vi "UIGetFlaggedRefs.vi"(6 "Check Flag (T)":bool=TRUE, 8 "error in":errorcluster, 10 "Flag":string, 11 "Control in":refnum<vi>) -> (0 "error out":errorcluster, 1 "UI Ctrl DataType":T1[](array[typedef]), 2 "UI Ctrl Names":string[](array[string]), 3 "UI Ctrl Refs":refnum<vi>[](array[refnum]))   [LabVIEW 2025, in "UI_Library.lvlib" / "UI_Library.lvclass"]
doc: "Get Control and subControls info"
uses:
  UI_Library.lvclass
  <vilib>/Utility/Data Type/Type Definitions/Data Type.ctl
  <vilib>/Utility/Data Type/NI_Data Type.lvlib
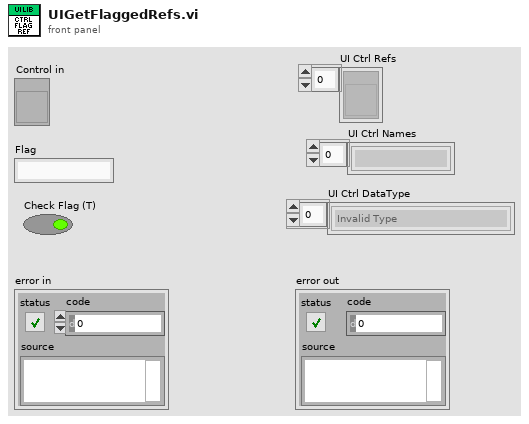
[diagram p1: front panel]
types:
  T1 = typedef "NI_Data Type.lvlib/Data Type.ctl" = enum8{"Invalid Type", "Void", "I8", "I16", "I32", "I64", "U8", "U16", "U32", "U64", "Single Float", "Double Float", "Extended Float", "Single Complex", "Double Complex", "Extended Complex", "Enum U8", "Enum U16", "Enum U32", "Enum U64", "Single Float With Unit", "Double Float With Unit", "Extended Float With Unit", "Single Complex with Unit", "Double Complex with Unit", "Extended Complex with Unit", "Boolean", "String", "Path", "Picture", "Tag", "Array", "Cluster", "Variant", "LV Variant", "Waveform", "Timestamp", "Digital Waveform", "Digital Data", "ExpressData", "Refnum", "External Data", "VI", "Poly VI", "LabVIEW Class Instance", "Fixed Point", "Set Collection", "Map Collection"}
  T2 = typedef "UI_Library.lvlib/UI_RefCluster.ctl" = cluster{"UI Ctrl Names":string[], "UI Ctrl DataType":T1[], "UI Ctrl Refs":refnum<vi>[]}
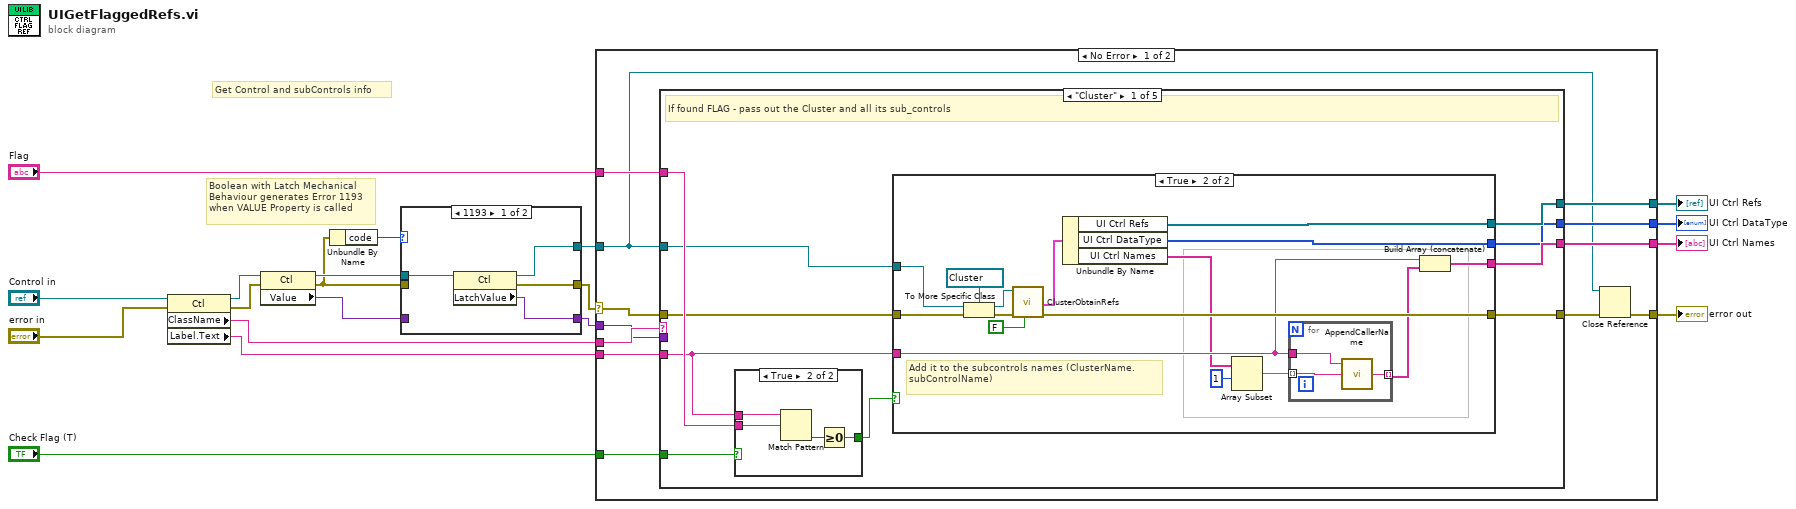
[diagram p0: block diagram]
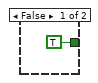
[diagram p3: hidden frame]
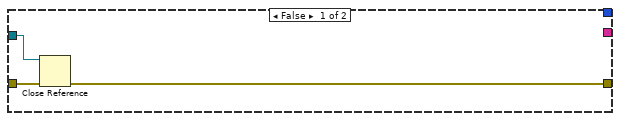
[diagram p4: hidden frame]
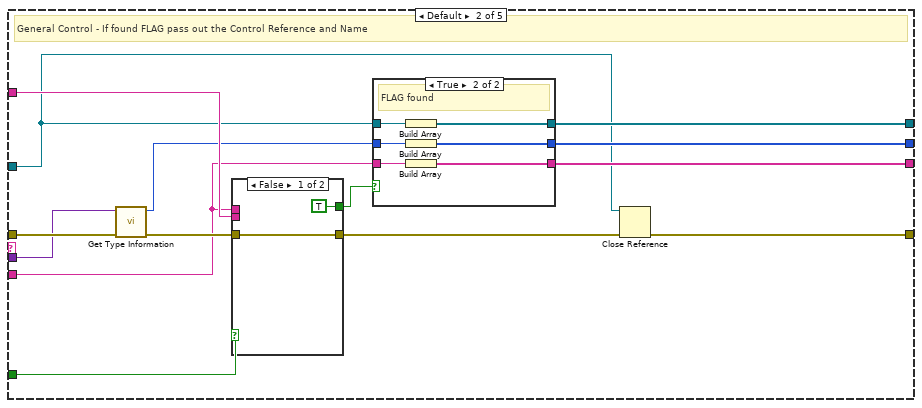
[diagram p5: hidden frame]
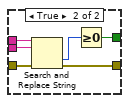
[diagram p6: hidden frame]
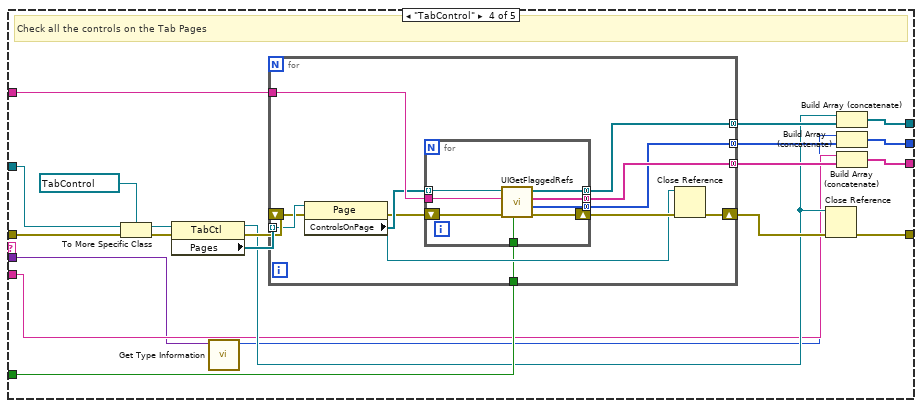
[diagram p9: hidden frame]
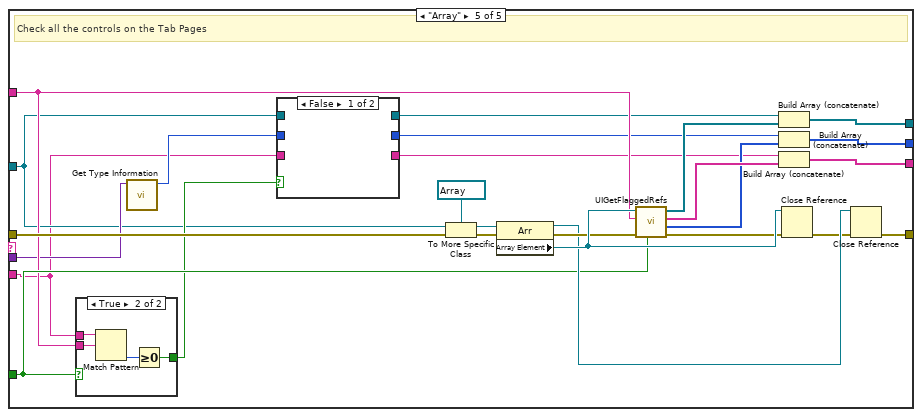
[diagram p10: hidden frame]
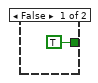
[diagram p12: hidden frame]
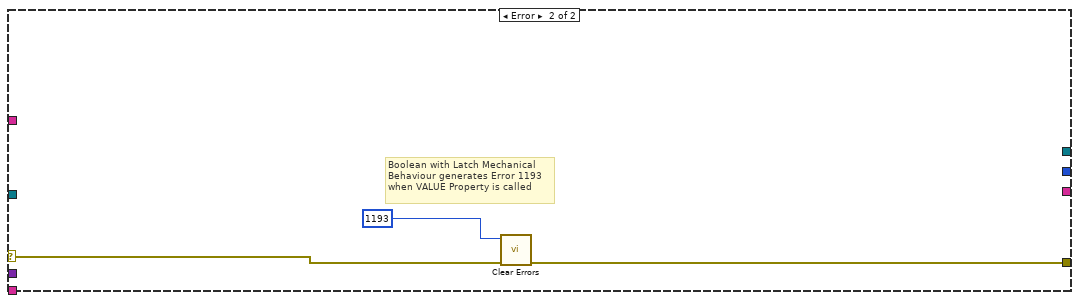
[diagram p13: hidden frame]
diagram:
  # "Get Control and subControls info"
  # "Boolean with Latch Mechanical\nBehaviour generates Error 1193 \nwhen VALUE Property is called"
  n1 = property on="Property Node" class="Ctl"(reference="Control in", error in="error in") -> (reference out=w8:refnum<vi>, error out=w9:errorcluster, "ClassName"=w16:string, "Label.Text"=w11:string)
  n2 = property on="Property Node" class="Ctl"(reference=w8, error in=w9) -> (reference out=w5:refnum<vi>, error out=w4:errorcluster, "Value"=w1:variant)
  n3 = Unbundle By Name(w4) -> ("code"=w7:i32)
  n4 = case shown="1193" w7 {
    tunnel: [w23 w25] -> w6
    tunnel: w5 -> [w22 w25]
    tunnel: w4 -> [_ w26]
    tunnel: [w21 w26] -> w3
    tunnel: [w20 w24] -> w2
    tunnel: w1 -> [_ w24]
    frame 1193 {
      n5 = property on="Property Node" class="Ctl"(reference=w22) -> (reference out=w23:refnum<vi>, error out=w21:errorcluster, "LatchValue"=w20:variant)  [unwired: 1 in]
    }
    frame Default {
    }
  }
  n6 = case shown="No Error" w3 {
    selector: w3 -> [w31 w182]
    tunnel: [w38 _] -> w19
    tunnel: [w37 _] -> w18
    tunnel: [w29 w180] -> w17
    tunnel: w16 -> [w36 _]
    tunnel: "Flag" -> [w35 _]
    tunnel: w6 -> [w28 _]
    tunnel: [w34 _] -> w12
    tunnel: w11 -> [w33 _]
    tunnel: w2 -> [w32 _]
    tunnel: "Check Flag (T)" -> [w27 _]
    frame No Error {
      n7 = case shown="\"Cluster\"" w36 {
        tunnel: w28 -> [w46 w78 _ w123 w151]
        tunnel: w33 -> [w40 w77 _ w107 w147]
        tunnel: [w44 w89 _ w111 w155] -> w38
        tunnel: [w43 w88 _ w108 w153] -> w37
        tunnel: w35 -> [w48 w86 _ w124 w157]
        tunnel: w31 -> [w45 w87 w104 w121 w169]
        tunnel: [w42 w80 w104 w113 w162] -> w30
        tunnel: [w41 w81 _ w109 w154] -> w34
        tunnel: w32 -> [_ w83 _ w105 w156]
        tunnel: w27 -> [w39 w76 _ w112 w158]
        frame "Cluster" {
          # "If found FLAG - pass out the Cluster and all its sub_controls"
          n8 = case shown="True" w39 {
            tunnel: w48 -> [_ w53]
            tunnel: [TRUE w51] -> w47
            tunnel: w40 -> [_ w50]
            frame False {
            }
            frame True {
              n9 = Match Pattern(string=w50, regular expression=w53) -> (offset past match=w52:i32)  [unwired: 1 in, 3 out]
              n10 = Greater Or Equal To 0?(x=w52) -> (x >= 0?=w51:bool)
            }
          }
          n11 = case shown="True" w47 {
            tunnel: w46 -> [w54 w69]
            tunnel: w45 -> [w56 w68]
            tunnel: [_ w66] -> w44
            tunnel: [_ w60] -> w43
            tunnel: [w55 w65] -> w42
            tunnel: w40 -> [_ w59]
            tunnel: [_ w57] -> w41
            frame False {
              n12 = Close Reference(reference=w54, error in (no error)=w56) -> (error out=w55:errorcluster)
            }
            frame True {
              # "Add it to the subcontrols names (ClusterName.subControlName)"
              n13 = To More Specific Class(target class=refnum<vi> refnum ("General Cluster Ref"), reference=w69, error in=w68) -> (specific class reference=w71:refnum<vi>, error out=w67:errorcluster)
              n14 = call "ClusterObtainRefs.vi"("Add Cluster Name?"=FALSE, "error in (no error)"=w67, "Clust Refnum"=w71) -> ("error out"=w65:errorcluster, "Ref cluster"=w72:T2)  [unwired: 7 in]
              n15 = Unbundle By Name(w72) -> ("UI Ctrl Refs"=w66:refnum<vi>[], "UI Ctrl DataType"=w57:T1[], "UI Ctrl Names"=w58:string[])
              n16 = Array Subset(array=w58, index=1) -> (w63:string[])  [unwired: 1 in]
              n17 = for {
                tunnel: w63 -> [w74] mode=indexing
                tunnel: w59 -> [w75]
                tunnel: [w73] -> w61 mode=indexing
                n18 = call "AppendCallerName.vi"("B"=w74, "A"=w75) -> ("A.B"=w73:string)  [unwired: 1 in]
              }
              n19 = Build Array (concatenate)(w59, w61) -> (w60:string[])
            }
          }
        }
        frame Default {
          # "General Control - If found FLAG pass out the Control Reference and Name"
          n20 = call <vilib>:"Get Type Information.vi"("error in (no error)"=w87, "variant"=w83) -> ("error out"=w84:errorcluster, "type"=w82:T1)  [unwired: 5 in, 3 out]
          n21 = case shown="False" w76 {
            tunnel: w86 -> [_ w96]
            tunnel: [TRUE w95] -> w85
            tunnel: w84 -> [w91 w94]
            tunnel: [w91 w93] -> w79
            tunnel: w77 -> [_ w92]
            frame False {
            }
            frame True {
              n22 = Search and Replace String(input string=w92, search string=w96, error in=w94) -> (offset past replacement=w97:i32, error out=w93:errorcluster)  [unwired: 5 in, 2 out]
              n23 = Greater Or Equal To 0?(x=w97) -> (x >= 0?=w95:bool)
            }
          }
          n24 = case shown="True" w85 {
            tunnel: w78 -> [_ w100]
            tunnel: [_ w103] -> w89
            tunnel: [_ w102] -> w88
            tunnel: w77 -> [_ w101]
            tunnel: w82 -> [_ w99]
            tunnel: [_ w98] -> w81
            frame False {
              # "FLAG Not Found"
            }
            frame True {
              # "FLAG found"
              n25 = Build Array(w100) -> (w103:refnum<vi>[])
              n26 = Build Array(w99) -> (w98:T1[])
              n27 = Build Array(w101) -> (w102:string[])
            }
          }
          n28 = Close Reference(reference=w78, error in (no error)=w79) -> (error out=w80:errorcluster)
        }
        frame "" {
          # "UNKNOWN Class Name"
        }
        frame "TabControl" {
          # "Check all the controls on the Tab Pages"
          n29 = To More Specific Class(target class=refnum<vi> refnum ("Tab Control"), reference=w123, error in=w121) -> (specific class reference=w119:refnum<vi>, error out=w120:errorcluster)
          n30 = property on="Property Node" class="TabCtl"(reference=w119, error in=w120) -> (reference out=w110:refnum<vi>, error out=w118:errorcluster, "Pages"=w125:refnum<vi>[])
          n31 = call <vilib>:"Get Type Information.vi"("variant"=w105) -> ("type"=w106:T1)  [unwired: 6 in, 4 out]
          n32 = for {
            tunnel: w125 -> [w137] mode=indexing
            tunnel: w124 -> [w136]
            shift-right: [w129] -> w114
            shift-left: w118 -> [w135]
            tunnel: [w132] -> w117 mode=concatenating
            tunnel: [w131] -> w116 mode=concatenating
            tunnel: [w130] -> w115 mode=concatenating
            tunnel: w112 -> [w126]
            n33 = property on="Property Node" class="Page"(reference=w137, error in=w135) -> (reference out=w127:refnum<vi>, error out=w133:errorcluster, "ControlsOnPage"=w134:refnum<vi>[])
            n34 = for {
              tunnel: w136 -> [w145]
              tunnel: w134 -> [w144] mode=indexing
              tunnel: [w141] -> w132 mode=concatenating
              tunnel: [w140] -> w131 mode=concatenating
              shift-right: [w142] -> w128
              shift-left: w133 -> [w143]
              tunnel: [w139] -> w130 mode=concatenating
              tunnel: w126 -> [w138]
              n35 = call "UIGetFlaggedRefs.vi"("Check Flag (T)"=w138, "error in"=w143, "Flag"=w145, "Control in"=w144) -> ("error out"=w142:errorcluster, "UI Ctrl DataType"=w139:T1[], "UI Ctrl Names"=w141:string[], "UI Ctrl Refs"=w140:refnum<vi>[])  [unwired: 4 in]
            }
            n36 = Close Reference(reference=w127, error in (no error)=w128) -> (error out=w129:errorcluster)
          }
          n37 = Close Reference(reference=w110, error in (no error)=w114) -> (error out=w113:errorcluster)
          n38 = Build Array (concatenate)(w110, w116) -> (w111:refnum<vi>[])
          n39 = Build Array (concatenate)(w106, w115) -> (w109:T1[])
          n40 = Build Array (concatenate)(w107, w117) -> (w108:string[])
        }
        frame "Array" {
          # "Check all the controls on the Tab Pages"
          n41 = case shown="True" w158 {
            tunnel: w157 -> [_ w179]
            tunnel: [TRUE w177] -> w152
            tunnel: w147 -> [_ w176]
            frame False {
            }
            frame True {
              n42 = Match Pattern(string=w176, regular expression=w179) -> (offset past match=w178:i32)  [unwired: 1 in, 3 out]
              n43 = Greater Or Equal To 0?(x=w178) -> (x >= 0?=w177:bool)
            }
          }
          n44 = call <vilib>:"Get Type Information.vi"("variant"=w156) -> ("type"=w149:T1)  [unwired: 6 in, 4 out]
          n45 = case shown="False" w152 {
            tunnel: w151 -> [_ w174]
            tunnel: [_ w174] -> w150
            tunnel: w149 -> [_ w173]
            tunnel: [_ w173] -> w148
            tunnel: w147 -> [_ w172]
            tunnel: [_ w172] -> w146
            frame False {
            }
            frame True {
            }
          }
          n46 = To More Specific Class(target class=refnum<vi> refnum ("Tab Control"), reference=w151, error in=w169) -> (specific class reference=w167:refnum<vi>, error out=w168:errorcluster)
          n47 = property on="Property Node" class="Arr"(reference=w167, error in=w168) -> (reference out=w161:refnum<vi>, error out=w166:errorcluster, "Array Element"=w171:refnum<vi>)
          n48 = call "UIGetFlaggedRefs.vi"("Check Flag (T)"=w158, "error in"=w166, "Flag"=w157, "Control in"=w171) -> ("error out"=w159:errorcluster, "UI Ctrl DataType"=w163:T1[], "UI Ctrl Names"=w165:string[], "UI Ctrl Refs"=w164:refnum<vi>[])  [unwired: 4 in]
          n49 = Build Array (concatenate)(w150, w164) -> (w155:refnum<vi>[])
          n50 = Build Array (concatenate)(w148, w163) -> (w154:T1[])
          n51 = Build Array (concatenate)(w146, w165) -> (w153:string[])
          n52 = Close Reference(reference=w171, error in (no error)=w159) -> (error out=w160:errorcluster)
          n53 = Close Reference(reference=w161, error in (no error)=w160) -> (error out=w162:errorcluster)
        }
      }
      n54 = Close Reference(reference=w28, error in (no error)=w30) -> (error out=w29:errorcluster)
    }
    frame Error {
      # "Boolean with Latch Mechanical\nBehaviour generates Error 1193 \nwhen VALUE Property is called"
      n55 = call <vilib>:"Clear Errors.vi"("error in (no error)"=w182, "specific error code to clear (0: all)"=1193) -> ("error out"=w180:errorcluster)  [unwired: 4 in, 1 out]
    }
  }
  "UI Ctrl Refs" <- w19
  "UI Ctrl Names" <- w18
  "error out" <- w17
  "UI Ctrl DataType" <- w12
